vi "Expr_Event Select.vi"(7 "data string":string, 10 "错误输入（无错误）":errorcluster, 11 "event queue in":string[](array[string])) -> (2 "错误输出":errorcluster, 3 "event queue out":string[](array[string]))   [LabVIEW 2018]
uses:
  05.UserVI's/type defs/17x Audit Motion Data Seq Control.ctl
  05.UserVI's/type defs/17x AP Data Type.ctl
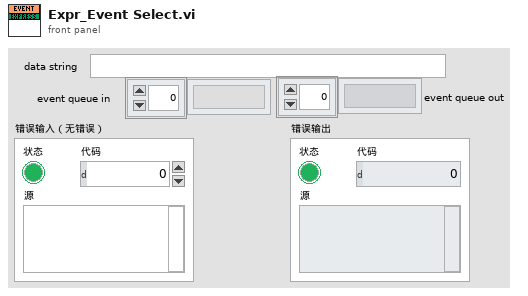
[diagram p1: front panel]
types:
  T1 = typedef "17x Audit Motion Data Seq Control.ctl" = cluster{"Power Supply Voltage":dbl, "Min Avg Current":dbl, "Max Avg Current":dbl, "Min Run Time":dbl, "Max Run Time":dbl, "Min Speed":dbl, "Max Speed":dbl, "AP Data % of Threshold":dbl, "Travel Distance":dbl, "AP Data Type":T2, "Check Current":bool, "Check Run Time":bool, "Check Speed":bool, "Express Motion?":bool, "Check Sound Test":bool, "Check Position?":bool, "Collect AP Data":bool, "Inital Position":u16, "End Position":u16, "Goto Posiition":u16, "Max max Current":dbl, "Min max Current":dbl, "Check max Current":bool, "Check Sound":bool, "Min Sound (dB)":dbl, "Max Sound (dB)":dbl, "SW Mode":enum16{"Hard Switch", "Uncond Frame"}, "LIN Msg":cluster{"ID":u8, "Msg":u8[][], "LDF":refnum<k21>}}
  T2 = typedef "17x AP Data Type.ctl" = enum16{"91/61", "92/62", "93/63", "67", "68", "6F", "71", "91 Msg", "92 Msg", "93 Msg", "94 Msg", "HiRain 91", "HiRain 92 Speed", "HiRain 92 HS", "HiRain 92", "HiRain 93", "SnT"}
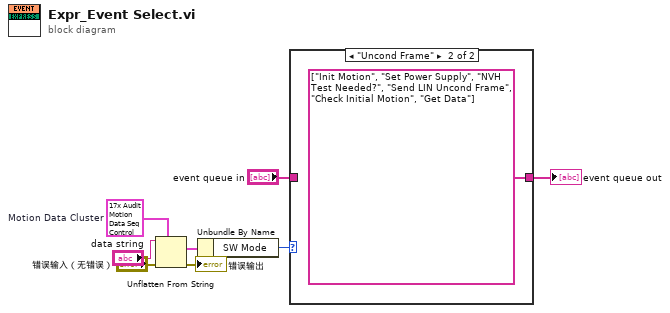
[diagram p0: block diagram]
diagram:
  w6 = T1 {"Power Supply Voltage"=0.0, "Min Avg Current"=0.0, "Max Avg Current"=0.0, "Min Run Time"=0.0, "Max Run Time"=0.0, "Min Speed"=0.0, "Max Speed"=0.0, "AP Data % of Threshold"=0.0, "Travel Distance"=0.0, "AP Data Type"=enum."91/61", "Check Current"=FALSE, "Check Run Time"=FALSE, "Check Speed"=FALSE, "Express Motion?"=FALSE, "Check Sound Test"=FALSE, "Check Position?"=FALSE, "Collect AP Data"=FALSE, "Inital Position"=0, "End Position"=0, "Goto Posiition"=0, "Max max Current"=0.0, "Min max Current"=0.0, "Check max Current"=FALSE, "Check Sound"=FALSE, "Min Sound (dB)"=0.0, "Max Sound (dB)"=0.0, "SW Mode"=enum."Hard Switch", "LIN Msg"={"ID"=0, "Msg"=[], "LDF"="EX1H"}}  # Motion Data Cluster
  n1 = Unflatten From String(type=w6, binary string="data string", error in (no error)="错误输入（无错误）") -> (value=w8:T1, error out=→"错误输出":errorcluster)  [unwired: 2 in, 1 out]
  n2 = Unbundle By Name(w8) -> ("SW Mode"=w7:enum16{"Hard Switch", "Uncond Frame"})
  n3 = case shown="\"Uncond Frame\"" w7 {
    tunnel: [w9 string[] ["Init Motion", "Set Power Supply", "NVH Test Needed?", "Send LIN Uncond Frame", "Check Initial Motion", "Get Data"] ("event queue out")] -> w4
    tunnel: "event queue in" -> [w9 _]
    frame "Hard Switch", Default {
    }
    frame "Uncond Frame" {
    }
  }
  "event queue out" <- w4
